vi "report results.vi"(8 "error in":errorcluster, 10 "result":refnum<class "result.lvclass">, 11 "actor reporter in":refnum<class "actor reporter.lvclass">) -> (0 "error out":errorcluster, 3 "actor reporter out":refnum<class "actor reporter.lvclass">)   [LabVIEW 2013, in "actor reporter.lvclass"]
uses:
  actor reporter.lvclass
  <vilib>/ActorFramework/Message Enqueuer/Message Enqueuer.lvclass
  actor message report/actor message report.lvclass
  result/result.lvclass
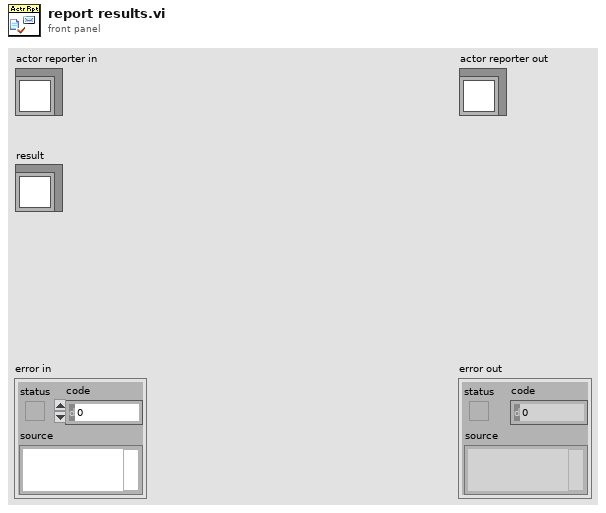
[diagram p1: front panel]
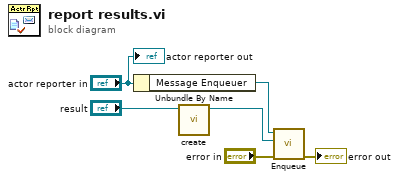
[diagram p0: block diagram]
diagram:
  n1 = Unbundle By Name("actor reporter in") -> ("Message Enqueuer"=w3:refnum<class "Message Enqueuer.lvclass">)
  n2 = call "create.vi"("result"="result") -> ("actor message report"=w1:refnum<class "actor message report.lvclass">)  [unwired: 10 in]
  n3 = call <vilib>:"Enqueue.vi"("error in (no error)"="error in", "Message"=w1, "Message Enqueuer in"=w3) -> ("error out"=→"error out":errorcluster)  [unwired: 7 in, 1 out]
  "actor reporter out" <- "actor reporter in"
